vi "Select_alarm.vi"(8 "Error in (no error)":errorcluster, 11 "Connection In":refnum<k7>) -> (0 "Historique alerte":string, 1 "Error out":errorcluster, 3 "Connection Out":refnum<k7>)   [LabVIEW 2019]
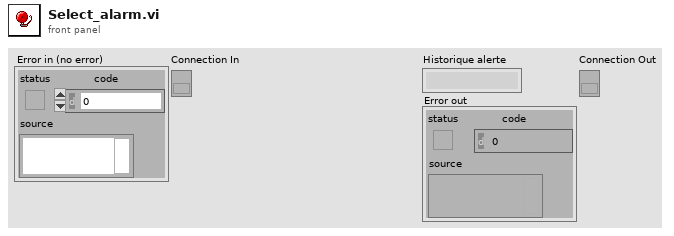
[diagram p1: front panel]
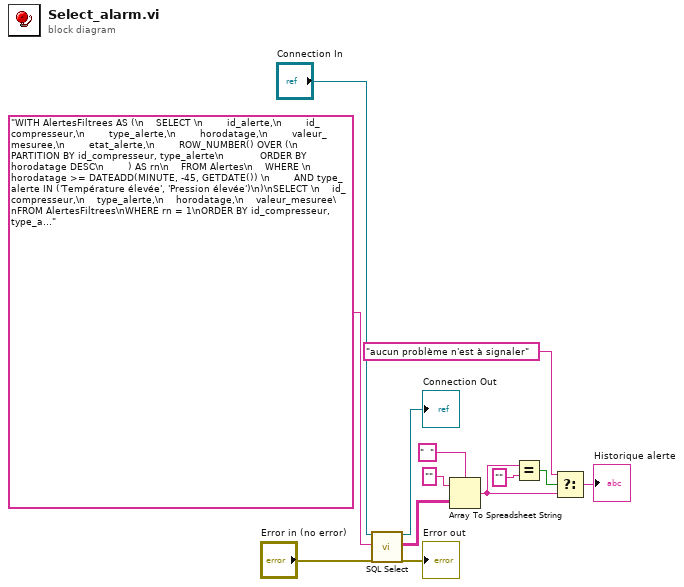
[diagram p0: block diagram]
diagram:
  n1 = call <vilib>:"SQL Select.vi"("Connection In"="Connection In", "SQL Query"="WITH AlertesFiltrees AS (\n    SELECT \n        id_alerte,\n        id_compresseur,\n        type_alerte,\n        horodatage,\n        valeur_mesuree,\n        etat_alerte,\n        ROW_NUMBER() OVER (\n            PARTITION BY id_compresseur, type_alerte\n            ORDER BY horodatage DESC\n        ) AS rn\n    FROM Alertes\n    WHERE \n        horodatage >= DATEADD(MINUTE, -45, GETDATE()) \n        AND type_alerte IN ('Température élevée', 'Pression élevée')\n)\nSELECT \n    id_compresseur,\n    type_alerte,\n    horodatage,\n    valeur_mesuree\nFROM AlertesFiltrees\nWHERE rn = 1\nORDER BY id_compresseur, type_alerte;\n", "Error in (no error)"="Error in (no error)") -> ("Connection Out"=→"Connection Out":refnum<k7>, "Data"=w10:string[][], "Error out"=→"Error out":errorcluster)  [unwired: 14 in]
  n2 = Array To Spreadsheet String(delimiter (Tab)="  ", array=w10, 3:"" ("format string")) -> (spreadsheet string=w3:string)
  n3 = Equal?(x=w3, y="") -> (x = y?=w4:bool)
  n4 = Select(t="aucun problème n'est à signaler", s=w4, f=w3) -> (s? t:f=→"Historique alerte":string)
